vi "CIE-Options Dialog.vi"(0 "Override smoothing":T2={"Speaker"=enum."Right primary", "Stimulus"={"Min Freq (Hz)"=50.0, "Max Freq (Hz)"=50000.0, "Freq Step (Hz)"=50.0, "Waveform"=enum."Chirp", "Attenuation (dB)"=20.0, "Sample Rate (Hz)"=100000.0}, "Averages"=0, "Left gain"=0.0, "Right gain"=0.0, "plot max"=FALSE, "smooth override"=FALSE, "Weighted"={"Folder"=path "", "Fmin"=0.0, "Fmax"=0.0, "Max range"=0.0, "WF"=0}, "Max Vmic"=0.0} {"Weighted"."WF" items=["Chirp", "Noise"]}) -> (4 "Override Out":T2={"Speaker"=enum."Right primary", "Stimulus"={"Min Freq (Hz)"=50.0, "Max Freq (Hz)"=50000.0, "Freq Step (Hz)"=50.0, "Waveform"=enum."Chirp", "Attenuation (dB)"=20.0, "Sample Rate (Hz)"=100000.0}, "Averages"=0, "Left gain"=0.0, "Right gain"=0.0, "plot max"=FALSE, "smooth override"=FALSE, "Weighted"={"Folder"=path "", "Fmin"=0.0, "Fmax"=0.0, "Max range"=0.0, "WF"=0}, "Max Vmic"=0.0} {"Weighted"."WF" items=["Chirp", "Noise"]}, 8 "Canceled?":bool)   [LabVIEW 2020]
uses:
  Type Defs/ACal-In Ear Parameters.ctl
  Utility VIs/Type Defs/Speaker ring.ctl
  Type Defs/Cal Stimulus.ctl
  Type Defs/ACal-Multiband Parameters.ctl
  Utility VIs/Buttons/KCheckmarkBoolean 2.ctl
panel:
  in  "Max Vmic":dbl caption="Maximum mic voltage" min=0.0 max=10.0
  in  "Apply smoothing?":T1 caption="Apply smoothing"
  in  "Cancel":bool
  in  "OK":bool
  # "In-Ear Calibration Options"
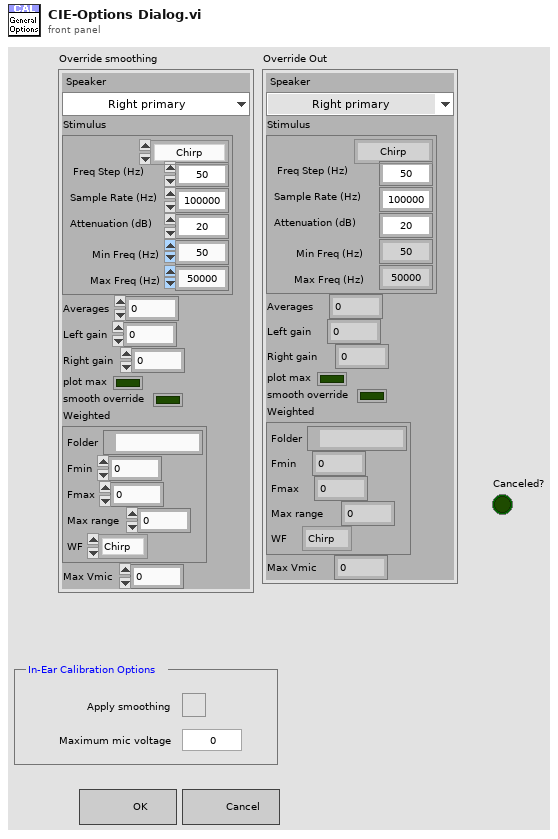
[diagram p1: front panel]
types:
  T1 = typedef "KCheckmarkBoolean 2.ctl" = bool
  T2 = typedef "ACal-In Ear Parameters.ctl" = cluster{"Speaker":T3, "Stimulus":T4, "Averages":i32, "Left gain":dbl, "Right gain":dbl, "plot max":bool, "smooth override":bool, "Weighted":T5, "Max Vmic":dbl}
  T3 = typedef "Speaker ring.ctl" = enum16{"Right primary", "Right secondary", "Left primary", "Left secondary"}
  T4 = typedef "Cal Stimulus.ctl" = cluster{"Min Freq (Hz)":dbl, "Max Freq (Hz)":dbl, "Freq Step (Hz)":dbl, "Waveform":enum16{"Chirp", "Weighted"}, "Attenuation (dB)":dbl, "Sample Rate (Hz)":dbl}
  T5 = typedef "ACal-Multiband Parameters.ctl" = cluster{"Folder":path, "Fmin":dbl, "Fmax":dbl, "Max range":dbl, "WF":u16}
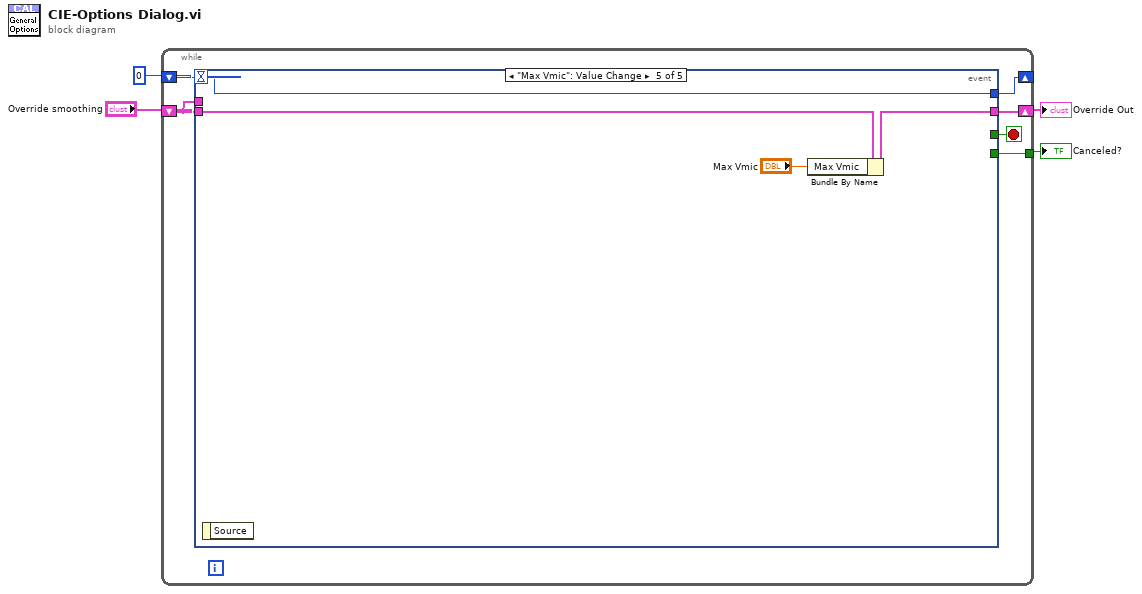
[diagram p0: block diagram]
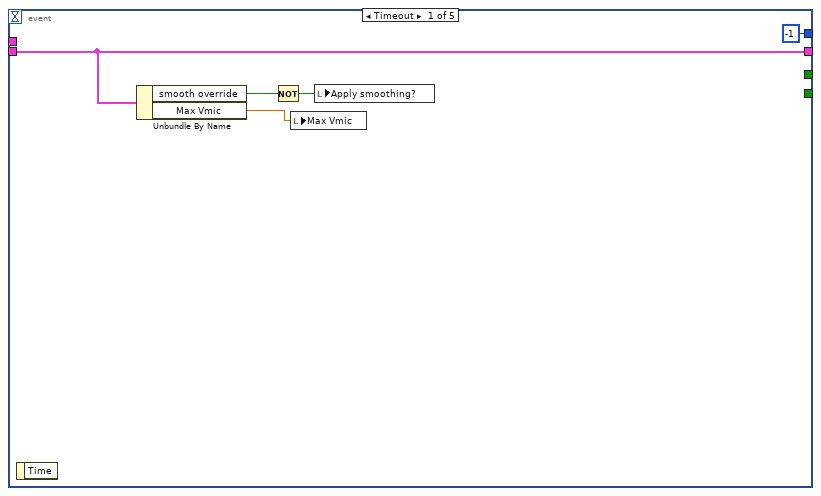
[diagram p2: hidden frame]
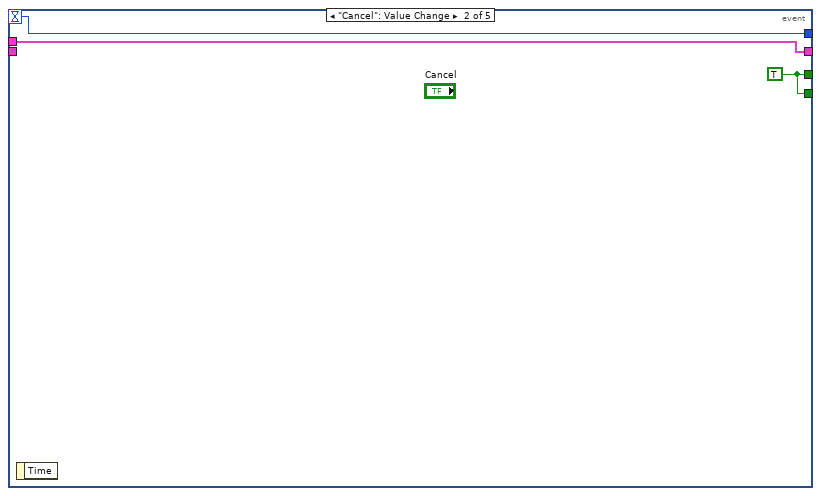
[diagram p3: hidden frame]
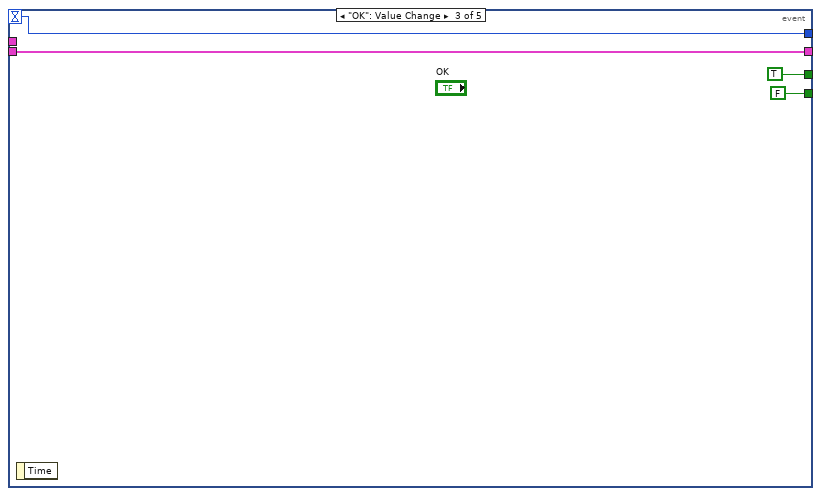
[diagram p4: hidden frame]
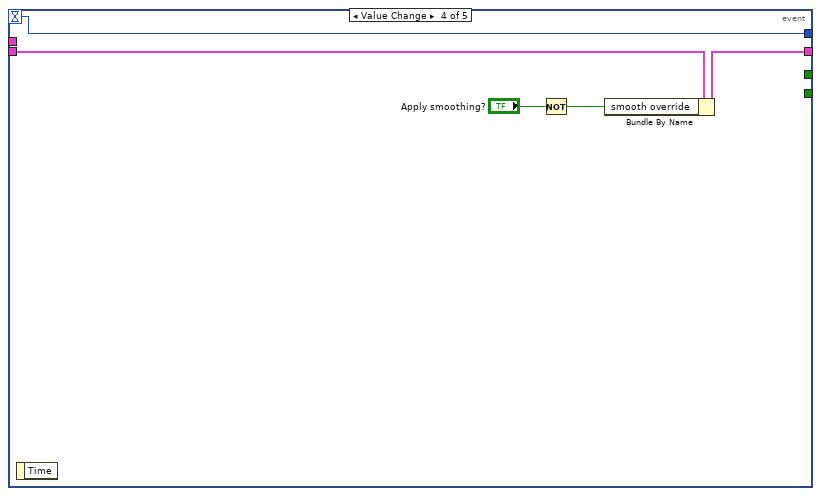
[diagram p5: hidden frame]
diagram:
  n1 = while {
    shift-right: [w9] -> _
    shift-left: 0 -> [w10]
    tunnel: [w6] -> w1
    shift-right: [w8] -> w2
    shift-left: "Override smoothing" -> [w5]
    stop <- w7 stop-if-true
    n2 = event shown="[4] \"Max Vmic\": Value Change" {
      selector: _ -> [_ _ _ _ _]
      dyn-events: _ -> [_ _ _ _ _]
      timeout: w10 -> [_ w18 w21 w26 w31]
      tunnel: [-1 w18 w21 w26 w31] -> w9
      tunnel: w5 -> [w13 _ w22 w25 w30]
      tunnel: [w13 w16 w22 w24 w29] -> w8
      tunnel: [_ w17 TRUE _ _] -> w7
      tunnel: [_ w17 FALSE _ _] -> w6
      tunnel: w5 -> [_ w16 _ _ _]
      event Timeout {
        n3 = event-data() -> ()  [unwired: 1 in, 1 out]
        n4 = Unbundle By Name(w13) -> ("smooth override"=w12:bool, "Max Vmic"=w11:dbl)
        n5 = Not(x=w12) -> (.not. x?=w14:bool)
        n6 = local write "Max Vmic"(w11) -> ()
        n7 = local write "Apply smoothing?"(w14) -> ()
      }
      event "Cancel": Value Change {
        w17 = TRUE
        n8 = event-data() -> ()  [unwired: 1 in, 1 out]
      }
      event "OK": Value Change {
        n9 = event-data() -> ()  [unwired: 1 in, 1 out]
      }
      event Value Change {
        n10 = event-data() -> ()  [unwired: 1 in, 1 out]
        n11 = Not(x="Apply smoothing?") -> (.not. x?=w23:T1)
        n12 = Bundle By Name(cluster=w25, "smooth override"=w23) -> (w24:T2)
      }
      event "Max Vmic": Value Change {
        n13 = event-data() -> ()  [unwired: 1 in, 1 out]
        n14 = Bundle By Name(cluster=w30, "Max Vmic"="Max Vmic") -> (w29:T2)
      }
    }
  }
  "Override Out" <- w2
  "Canceled?" <- w1
